vi "FPGA_9505_Thruster_Current_Loop.vi"() -> ()   [LabVIEW 2012]
uses:
  <vilib>/LabVIEW Targets/FPGA/cRIO/cRIO-9505/controls.llb/_nicrio_cRIO-9505_DriveStatus.ctl
  <vilib>/Platform/TimedLoop/XDataNode/timing_clust.ctl
  <vilib>/Platform/TimedLoop/XDataNode/nitl_modes.ctl
  <vilib>/Platform/TimedLoop/XDataNode/wakeup.ctl
  <vilib>/LabVIEW Targets/FPGA/cRIO/cRIO-9505/controls.llb/_nicrio_cRIO-9505_DriveDirection.ctl
  <vilib>/rvi/Emulation/niFpgaSctlEmulationRegisterWithScheduler.vi
  <vilib>/rvi/Emulation/niFpgaSctlEmulationScheduler.vi
  <vilib>/rvi/Emulation/niFpgaSctlEmulationGetInTimedLoop.vi
  <vilib>/rvi/eio/common/nirviEmuTemplateMethod_errors.vi
  <vilib>/rvi/Emulation/niFpgaSctlEmulationGlobalWrite.vi
  <vilib>/rvi/eio/common/nirviEmuTemplatePropertyGet_noerrors.vi
  <vilib>/Platform/TimedLoop/XDataNode/XDataNode.xnode
  <vilib>/eio/EIONode/EIONode.xnode
  <vilib>/eio/EIOMethodNode/EIOMethodNode.xnode
  <vilib>/eio/EIOPropertyNode/EIOPropertyNode.xnode
  <vilib>/rvi/eio/common/nirviEmuTemplatePropertyGet_errors.vi
  <vilib>/rvi/eio/common/nirviEmuTemplatePropertySet_errors.vi
  <vilib>/rvi/eio/common/nirviEmuTemplatePropertySet_noerrors.vi
  <vilib>/Platform/TimedLoop/XDataNode/XDNodeRunTimeDep.lvlib
panel:
  in  "Tab Control":enum32{"Control", "Debugging 1", "Debugging 2"}(tab)
  out "PWM Duty Cycle 3":i16
  in  "Current Loop\nRate (usec) 1":u32=50
  in  "Current Setpoint 1":i16 caption="Setpoint"
  in  "Current Limit 1":i16 caption="Setpoint"
  in  "Current Feedback 1":i16
  in  "Current PI gains 1":T1={"Proportional Gain"=20, "Integral Gain"=10, "Derivative Gain"=0}
  out "PWM Duty Cycle 4":i16
  in  "Current Loop\nRate (usec) 2":u32=50
  in  "Current Setpoint 2":i16 caption="Setpoint"
  in  "Current Limit 2":i16 caption="Setpoint"
  in  "Current Feedback 2":i16
  in  "Current PI gains 2":T1={"Proportional Gain"=20, "Integral Gain"=10, "Derivative Gain"=0}
  out "PWM Loop Counter 1":i32(graph)
  out "Sample Current Loop Counter 1":i32(graph)
  out "Current Sense 1":i16(graph)
  in  "Trig AI 1":bool
  out "PWM Duty Cycle 1":i16(graph)
  out "Current Loop Counter 1":i32(graph)
  out "PWM Loop Counter 2":i32(graph)
  out "PWM Duty Cycle 2":i16(graph)
  out "Current Loop Counter 2":i32(graph)
  in  "Trig AI 2":bool
  out "Current Sense 2":i16(graph)
  out "Sample Current Loop Counter 2":i32(graph)
  out "Vsup Present 2":bool
  out "Drive Fault 2":bool
  out "Drive Status 2":T2
  out "Temp Fault 2":bool
  in  "Enable\nDrive 2":bool
  in  "Disable\nDrive 2":bool
  out "Vsup Present 1":bool
  out "Drive Fault 1":bool
  out "Drive Status 1":T2
  out "Temp Fault 1":bool
  in  "Enable\nDrive 1":bool
  in  "Disable\nDrive 1":bool
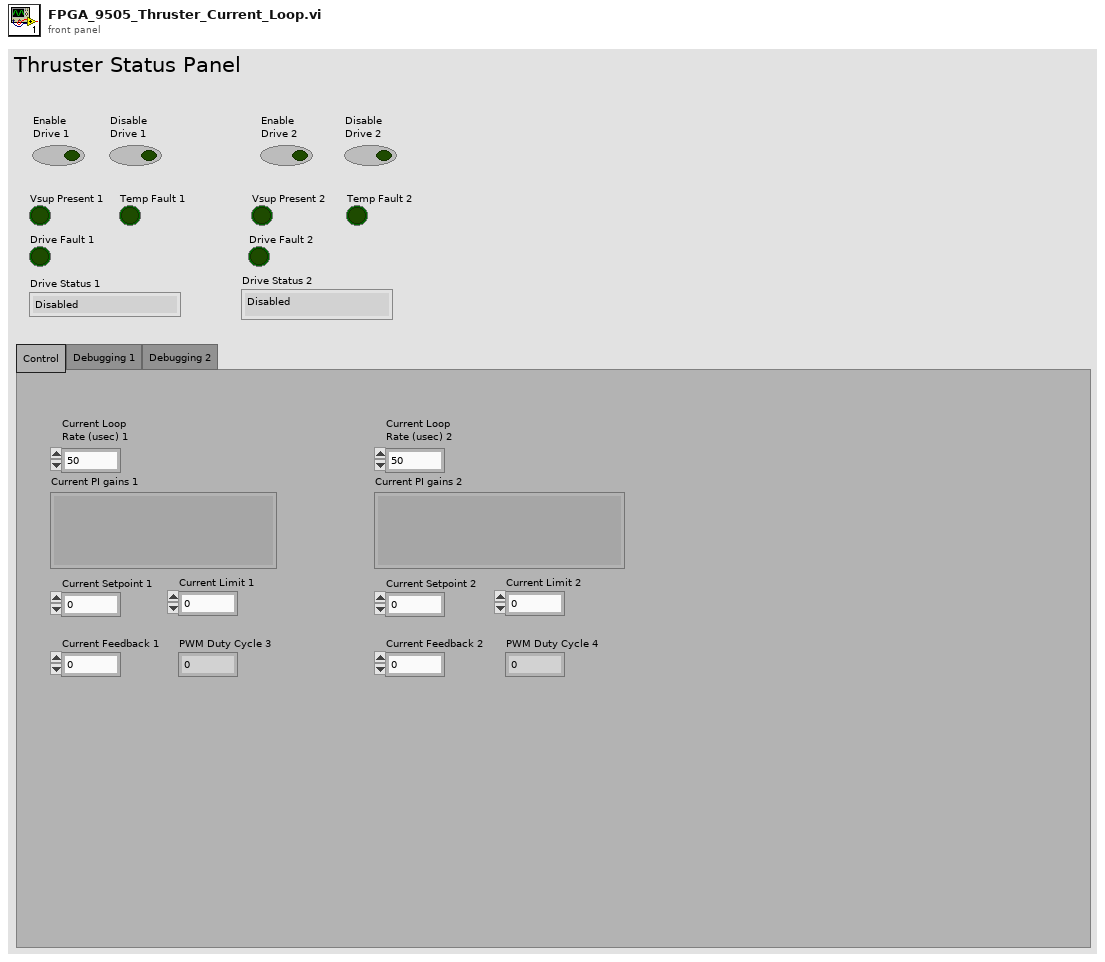
[diagram p1: front panel]
types:
  T1 = cluster{"Proportional Gain":i16, "Integral Gain":i16, "Derivative Gain":i16}
  T2 = typedef "_nicrio_cRIO-9505_DriveStatus.ctl" = enum8{"Enabled", "Disabled", "Disabled by Drive Fault", "Disabled by Temp. Fault", "Disabled by E-Stop", "Unknown"}
  T3 = typedef "XDNodeRunTimeDep.lvlib/timing_clust.ctl" = cluster{"Expected End [f-1]":u64, "Actual End [f-1]":u64, "Finished Late? [f-1]":bool, "Expected End [i-1]":u64, "Actual End [i-1]":u64, "Finished Late? [i-1]":bool, "Expected Start [i]":u64, "Actual Start [i]":u64, "Expected Start [f]":u64, "Actual Start [f]":u64, "Source Name":string, "Structure Name":string, "Period":i64, "Deadline":i64, "Offset":i64, "Start":i64, "Priority":i32, "Timeout":i32, "Mode":T4, "Wakeup Reason":T5, "Error":errorcluster, "Source Type":string, "Secondary Source Type":string, "Global End Time":u64, "Global Start Time":u64, "Frame Duration":u64, "Iteration Duration":u64, "Assigned CPU":i32, "I/O Scan Engine Mode":u32}
  T4 = typedef "XDNodeRunTimeDep.lvlib/nitl_modes.ctl" = enum32{"No Change", "Process missed periods, maintain original phase", "Discard missed periods, maintain original phase", "Process missed periods, ignore original phase", "Discard missed periods, ignore original phase"}
  T5 = typedef "XDNodeRunTimeDep.lvlib/wakeup.ctl" = enum32{"Normal", "Aborted", "Asynchronous wakeup", "Timing source error", "Timed loop error", "Timeout"}
  T6 = typedef "_nicrio_cRIO-9505_DriveDirection.ctl" = enum8{"Clockwise", "Counterclockwise"}
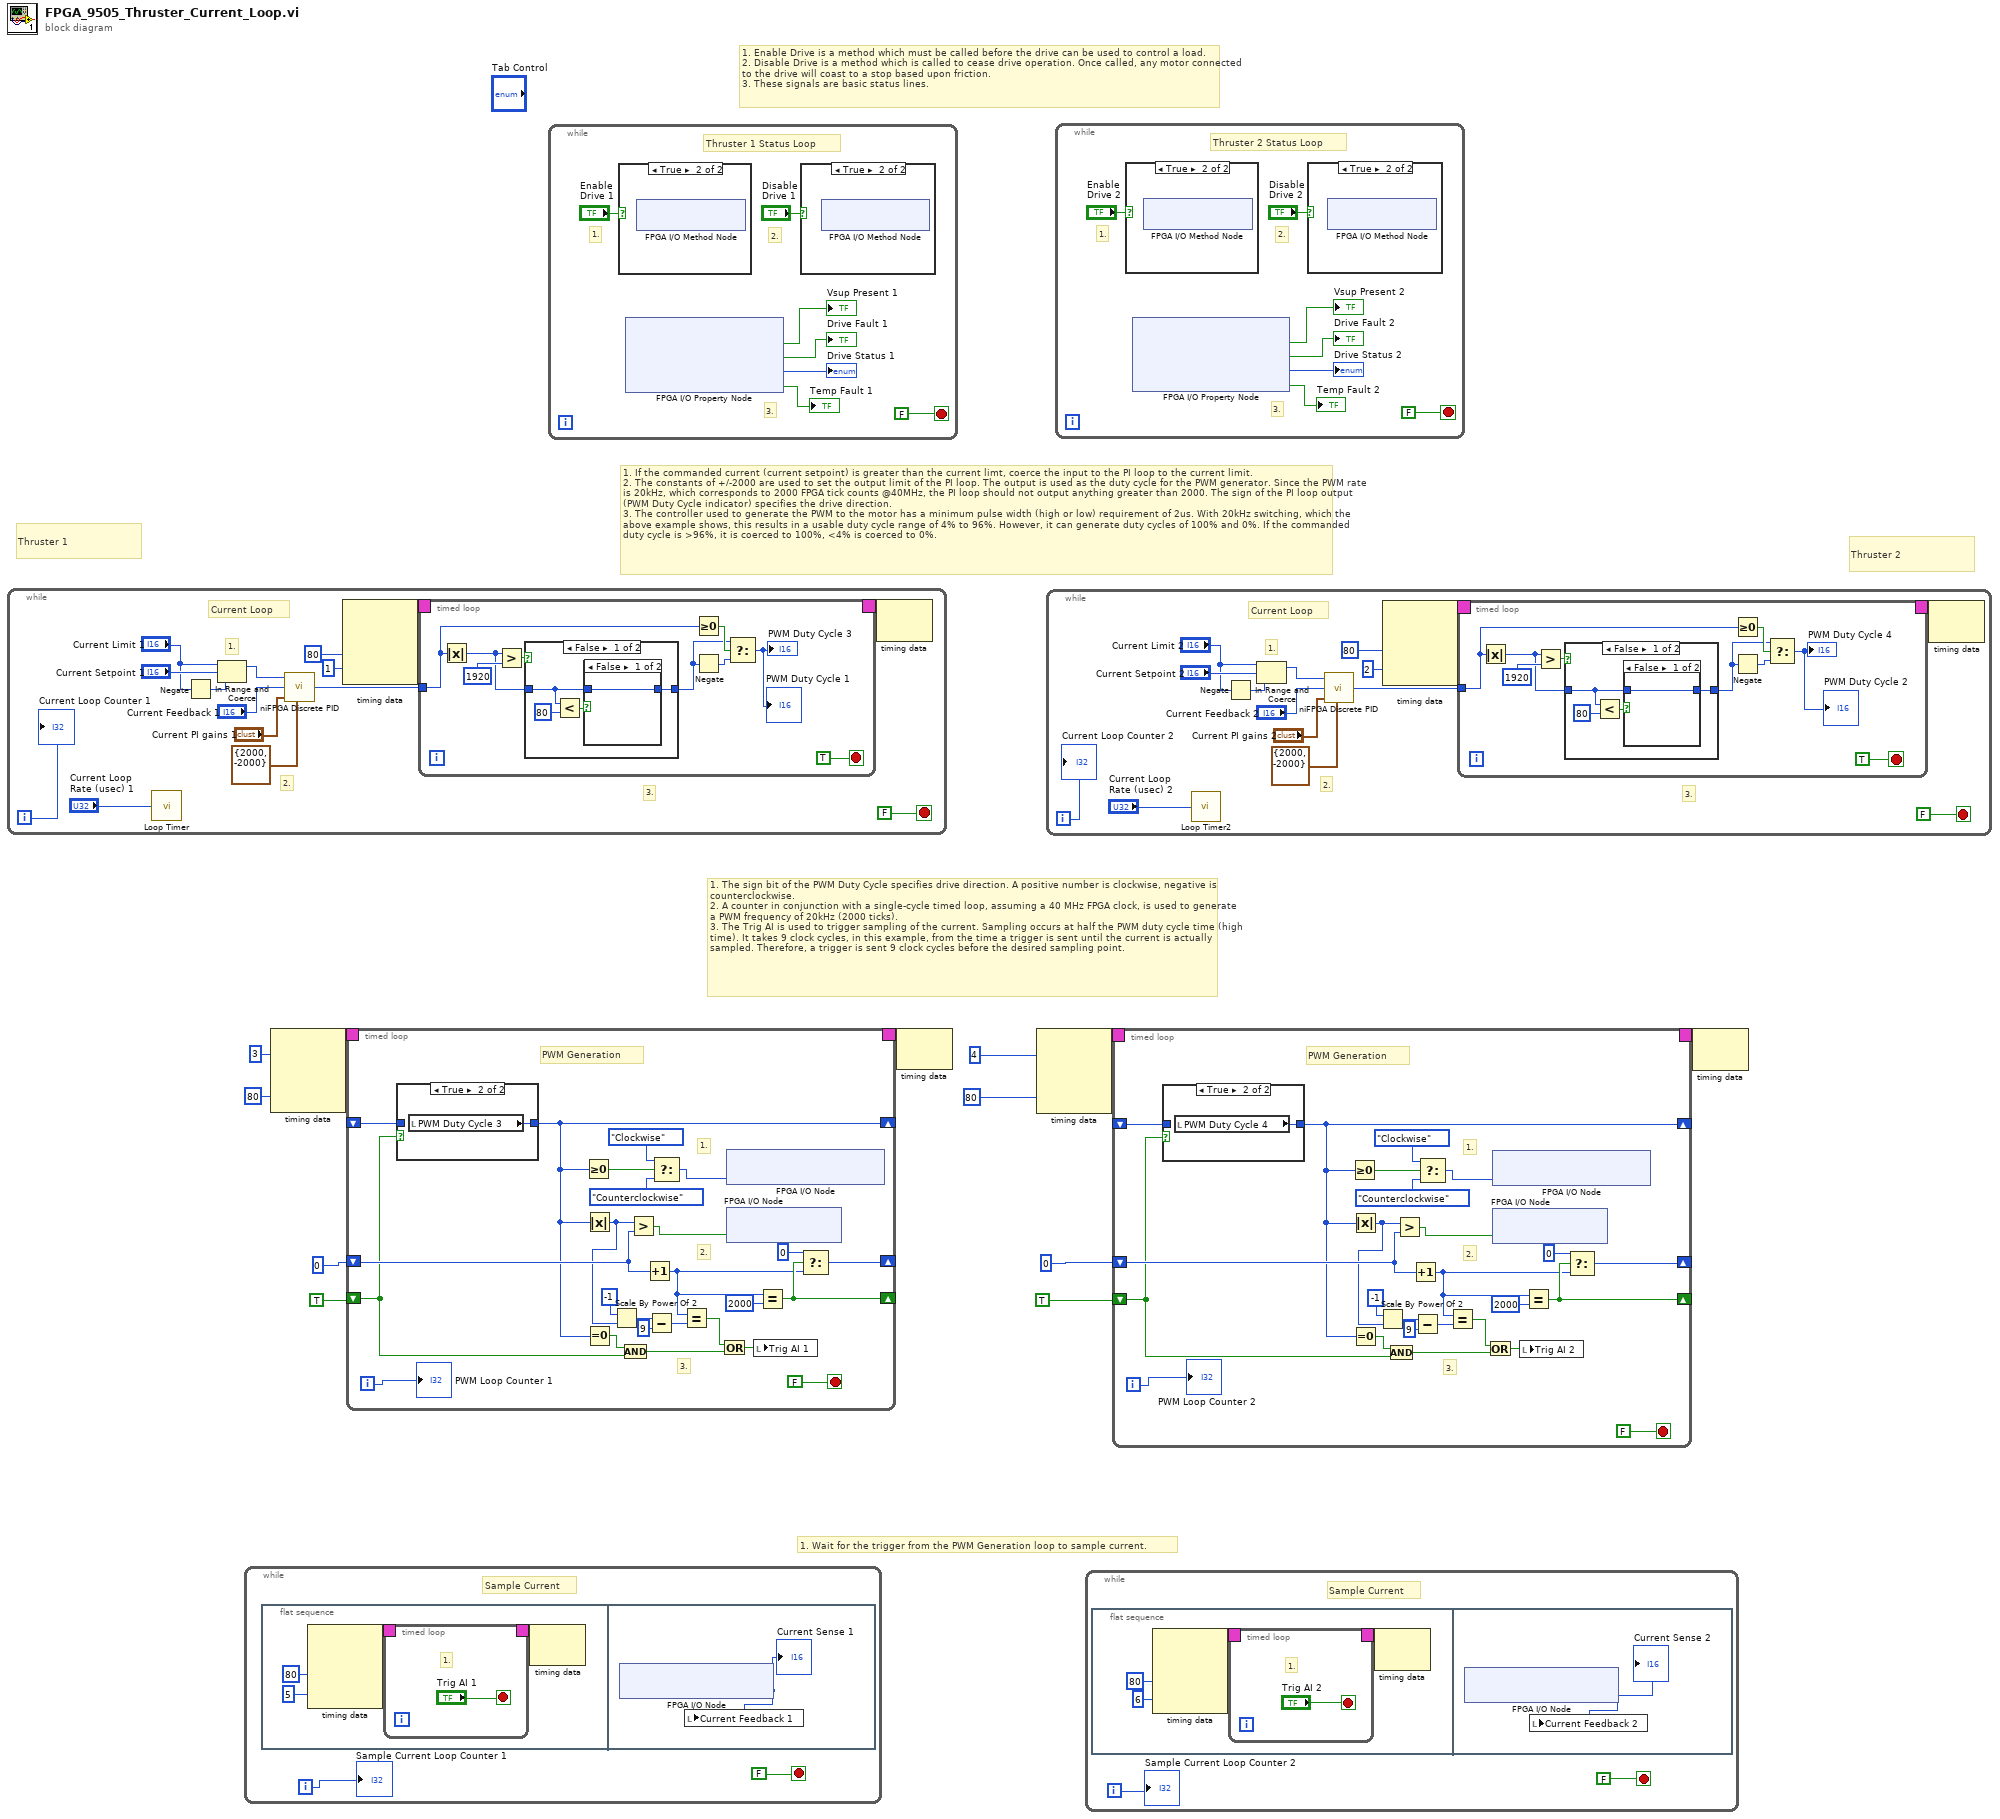
[diagram p0: block diagram]
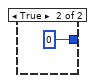
[diagram p4: hidden frame]
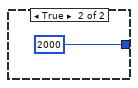
[diagram p5: hidden frame]
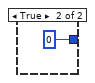
[diagram p6: hidden frame]
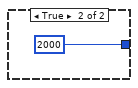
[diagram p7: hidden frame]
diagram:
  # "1. Wait for the trigger from the PWM Generation loop to sample current."
  # "1. The sign bit of the PWM Duty Cycle specifies drive direction. A positive number is clockwise, negative is counterclockwise.\n2. A counter in conjunction with a single-cycle timed loop, assuming a 40 MHz FPGA clock, is used to generate a PWM frequency of 20kHz (2000 ticks).\n3. The Trig AI is used to trigger sampling of the current. Sampling occurs at half the PWM duty cycle time (high time). It takes 9 clock cycles, in this example, from the time a trigger is sent until the current is actually sampled. Therefore, a trigger is sent 9 clock cycles before the desired sampling point."
  # "1. If the commanded current (current setpoint) is greater than the current limt, coerce the input to the PI loop to the current limit.\n2. The constants of +/-2000 are used to set the output limit of the PI loop. The output is used as the duty cycle for the PWM generator. Since the PWM rate is 20kHz, which corresponds to 2000 FPGA tick counts @40MHz, the PI loop should not output anything greater than 2000. The sign of the PI loop output (PWM Duty Cycle indicator) specifies the drive direction.\n3. The controller used to generate the PWM to the motor has a minimum pulse width (high or low) requirement of 2us. With 20kHz switching, which the above example shows, this results in a usable duty cycle range of 4% to 96%. However, it can generate duty cycles of 100% and 0%. If the commanded duty c..."
  # "Thruster 2"
  # "Thruster 1"
  # "1. Enable Drive is a method which must be called before the drive can be used to control a load.\n2. Disable Drive is a method which is called to cease drive operation. Once called, any motor connected to the drive will coast to a stop based upon friction.\n3. These signals are basic status lines."
  n1 = while {
    i -> [w15]
    stop <- FALSE stop-if-true
    # "3."
    # "2."
    # "1."
    # "Current Loop"
    n2 = call "Loop Timer"("Count(uSec)"="Current Loop\nRate (usec) 1") -> ()  [unwired: 1 out]
    n3 = Negate(x="Current Limit 1") -> (-x=w20:i16)
    n4 = In Range and Coerce(upper limit="Current Limit 1", x="Current Setpoint 1", lower limit=w20) -> (coerced(x)=w18:i16)  [unwired: 1 out]
    n5 = call <vilib>:"niFPGA Discrete PID.vi"("setpoint"=w18, "process variable"="Current Feedback 1", "PID gains (x 2^8)"="Current PI gains 1", "output range"=cluster{"output high":i16, "output low":i16} {"output high"=2000, "output low"=-2000}) -> ("output"=w24:i16)  [unwired: 1 in, 4 out]
    n6 = node-c288(80, 1) -> (w23:T3)  [unwired: 2 out]
    n7 = timed-loop {
      timing: w23 -> [_]
      timing-out: [_] -> w22
      tunnel: w24 -> [w30]
      stop <- TRUE stop-if-true
      n8 = Absolute Value(x=w30) -> (abs(x)=w31:i16)
      n9 = Greater?(x=w31, y=i16 1920) -> (0:w33:bool)
      n10 = case shown="False" w33 {
        tunnel: [w39 i16 2000] -> w32
        tunnel: w31 -> [w37 _]
        frame False {
          n11 = Less?(x=w37, y=i16 80) -> (x < y?=w38:bool)
          n12 = case shown="False" w38 {
            tunnel: [w41 i16 0] -> w39
            tunnel: w37 -> [w41 _]
            frame False {
            }
            frame True {
            }
          }
        }
        frame True {
        }
      }
      n13 = Greater Or Equal To 0?(x=w30) -> (x >= 0?=w36:bool)
      n14 = Negate(x=w32) -> (-x=w35:i16)
      n15 = Select(t=w32, s=w36, f=w35) -> (s? t:f=→"PWM Duty Cycle 3" →"PWM Duty Cycle 1":i16)
    }
    n16 = node-c288(w22) -> ()  [unwired: 1 out]
    "Current Loop Counter 1" <- w15
  }
  n17 = while {
    i -> [w51]
    stop <- FALSE stop-if-true
    # "Sample Current"
    n18 = flat-sequence {
      frame #0 {
        n19 = node-c288(80, 5) -> (w56:T3)  [unwired: 2 out]
        n20 = timed-loop {
          timing: w56 -> [_]
          timing-out: [_] -> w55
          stop <- "Trig AI 1" stop-if-true
          # "1."
        }
        n21 = node-c288(w55) -> ()  [unwired: 1 out]
      }
      frame #1 {
        n22 = xnode "FPGA I/O Node"() -> ("Mod2/Current Sense 2"=w65:i16)  [unwired: 1 in, 1 out]
        "Current Sense 1" <- w65
        n23 = local write "Current Feedback 1"(w65) -> ()
      }
    }
    "Sample Current Loop Counter 1" <- w51
  }
  n24 = node-c288(3, 80) -> (w12:T3)  [unwired: 2 in]
  n25 = timed-loop {
    timing: w12 -> [_]
    timing-out: [_] -> w11
    shift-right: [w87] -> _
    shift-left: i16 0 -> [w90]
    shift-right: [w86] -> _
    shift-left: TRUE -> [w83]
    shift-right: [w72] -> _
    shift-left: _ -> [w85]
    i -> [w66]
    stop <- FALSE stop-if-true
    # "3."
    # "2."
    # "1."
    # "PWM Generation"
    n26 = case shown="True" w83 {
      tunnel: [w91 w92] -> w72
      tunnel: w85 -> [w91 _]
      frame False {
      }
      frame True {
        n27 = local read "PWM Duty Cycle 3"() -> (w92:i16)
      }
    }
    n28 = Greater Or Equal To 0?(x=w72) -> (x >= 0?=w79:bool)
    n29 = Absolute Value(x=w72) -> (abs(x)=w70:i16)
    n30 = Equal To 0?(x=w72) -> (x = 0?=w84:bool)
    n31 = Scale By Power Of 2(n=i8 -1, x=w70) -> (x*2^n=w74:i16)
    n32 = And(x=w84, y=w83) -> (x .and. y?=w80:bool)
    n33 = Greater?(x=w70, y=w90) -> (0:w67:bool)
    n34 = Increment(x=w90) -> (x+1=w82:i16)
    n35 = Subtract(x=w74, y=i8 9) -> (x-y=w73:i16)
    n36 = Select(t=_nicrio_cRIO-9505_DriveDirection."Clockwise", s=w79, f=_nicrio_cRIO-9505_DriveDirection."Counterclockwise") -> (s? t:f=w68:T6)
    n37 = Equal?(x=w82, y=w73) -> (x = y?=w81:bool)
    n38 = Or(x=w81, y=w80) -> (x .or. y?=w76:bool)
    n39 = xnode "FPGA I/O Node"("Mod2/Drive Direction 2"=w68) -> ()  [unwired: 1 in, 1 out]
    n40 = xnode "FPGA I/O Node"("Mod2/Motor 2"=w67) -> ()  [unwired: 1 in, 1 out]
    n41 = local write "Trig AI 1"(w76) -> ()
    n42 = Equal?(x=w82, y=i16 2000) -> (x = y?=w86:bool)
    n43 = Select(t=i16 0, s=w86, f=w82) -> (s? t:f=w87:i16)
    "PWM Loop Counter 1" <- w66
  }
  n44 = while {
    stop <- FALSE stop-if-true
    # "3."
    # "2."
    # "1."
    # "Thruster 1 Status Loop"
    n45 = case shown="True" "Enable\nDrive 1" {
      frame False {
      }
      frame True {
        n46 = xnode "FPGA I/O Method Node"() -> ()  [unwired: 1 in, 1 out]
      }
    }
    n47 = xnode "FPGA I/O Property Node"() -> ("Vsup Present"=→"Vsup Present 1":bool, "Drive Fault"=→"Drive Fault 1":bool, "Drive Status"=→"Drive Status 1":T2, "Over Temperature Fault"=→"Temp Fault 1":bool)  [unwired: 1 in, 1 out]
    n48 = case shown="True" "Disable\nDrive 1" {
      frame False {
      }
      frame True {
        n49 = xnode "FPGA I/O Method Node"() -> ()  [unwired: 1 in, 1 out]
      }
    }
  }
  n50 = node-c288(w11) -> ()  [unwired: 1 out]
  n51 = node-c288(4, 80) -> (w6:T3)  [unwired: 2 in]
  n52 = while {
    i -> [w104]
    stop <- FALSE stop-if-true
    # "3."
    # "2."
    # "1."
    # "Current Loop"
    n53 = call "Loop Timer2"("Count(uSec)"="Current Loop\nRate (usec) 2") -> ()  [unwired: 1 out]
    n54 = Negate(x="Current Limit 2") -> (-x=w109:i16)
    n55 = In Range and Coerce(upper limit="Current Limit 2", x="Current Setpoint 2", lower limit=w109) -> (coerced(x)=w107:i16)  [unwired: 1 out]
    n56 = call <vilib>:"niFPGA Discrete PID.vi"("setpoint"=w107, "process variable"="Current Feedback 2", "PID gains (x 2^8)"="Current PI gains 2", "output range"=cluster{"output high":i16, "output low":i16} {"output high"=2000, "output low"=-2000}) -> ("output"=w113:i16)  [unwired: 1 in, 4 out]
    n57 = node-c288(80, 2) -> (w112:T3)  [unwired: 2 out]
    n58 = timed-loop {
      timing: w112 -> [_]
      timing-out: [_] -> w111
      tunnel: w113 -> [w119]
      stop <- TRUE stop-if-true
      n59 = Absolute Value(x=w119) -> (abs(x)=w120:i16)
      n60 = Greater?(x=w120, y=i16 1920) -> (0:w122:bool)
      n61 = case shown="False" w122 {
        tunnel: [w128 i16 2000] -> w121
        tunnel: w120 -> [w126 _]
        frame False {
          n62 = Less?(x=w126, y=i16 80) -> (x < y?=w127:bool)
          n63 = case shown="False" w127 {
            tunnel: [w130 i16 0] -> w128
            tunnel: w126 -> [w130 _]
            frame False {
            }
            frame True {
            }
          }
        }
        frame True {
        }
      }
      n64 = Greater Or Equal To 0?(x=w119) -> (x >= 0?=w125:bool)
      n65 = Negate(x=w121) -> (-x=w124:i16)
      n66 = Select(t=w121, s=w125, f=w124) -> (s? t:f=→"PWM Duty Cycle 4" →"PWM Duty Cycle 2":i16)
    }
    n67 = node-c288(w111) -> ()  [unwired: 1 out]
    "Current Loop Counter 2" <- w104
  }
  n68 = while {
    stop <- FALSE stop-if-true
    # "3."
    # "2."
    # "1."
    # "Thruster 2 Status Loop"
    n69 = case shown="True" "Enable\nDrive 2" {
      frame False {
      }
      frame True {
        n70 = xnode "FPGA I/O Method Node"() -> ()  [unwired: 1 in, 1 out]
      }
    }
    n71 = xnode "FPGA I/O Property Node"() -> ("Vsup Present"=→"Vsup Present 2":bool, "Drive Fault"=→"Drive Fault 2":bool, "Drive Status"=→"Drive Status 2":T2, "Over Temperature Fault"=→"Temp Fault 2":bool)  [unwired: 1 in, 1 out]
    n72 = case shown="True" "Disable\nDrive 2" {
      frame False {
      }
      frame True {
        n73 = xnode "FPGA I/O Method Node"() -> ()  [unwired: 1 in, 1 out]
      }
    }
  }
  n74 = while {
    i -> [w147]
    stop <- FALSE stop-if-true
    # "Sample Current"
    n75 = flat-sequence {
      frame #0 {
        n76 = node-c288(80, 6) -> (w152:T3)  [unwired: 2 out]
        n77 = timed-loop {
          timing: w152 -> [_]
          timing-out: [_] -> w151
          stop <- "Trig AI 2" stop-if-true
          # "1."
        }
        n78 = node-c288(w151) -> ()  [unwired: 1 out]
      }
      frame #1 {
        n79 = xnode "FPGA I/O Node"() -> ("Mod4/Current Sense 2"=w161:i16)  [unwired: 1 in, 1 out]
        "Current Sense 2" <- w161
        n80 = local write "Current Feedback 2"(w161) -> ()
      }
    }
    "Sample Current Loop Counter 2" <- w147
  }
  n81 = timed-loop {
    timing: w6 -> [_]
    timing-out: [_] -> w5
    shift-right: [w183] -> _
    shift-left: i16 0 -> [w186]
    shift-right: [w182] -> _
    shift-left: TRUE -> [w179]
    shift-right: [w168] -> _
    shift-left: _ -> [w181]
    i -> [w162]
    stop <- FALSE stop-if-true
    # "3."
    # "2."
    # "1."
    # "PWM Generation"
    n82 = case shown="True" w179 {
      tunnel: [w187 w188] -> w168
      tunnel: w181 -> [w187 _]
      frame False {
      }
      frame True {
        n83 = local read "PWM Duty Cycle 4"() -> (w188:i16)
      }
    }
    n84 = Greater Or Equal To 0?(x=w168) -> (x >= 0?=w175:bool)
    n85 = Absolute Value(x=w168) -> (abs(x)=w166:i16)
    n86 = Equal To 0?(x=w168) -> (x = 0?=w180:bool)
    n87 = Scale By Power Of 2(n=i8 -1, x=w166) -> (x*2^n=w170:i16)
    n88 = And(x=w180, y=w179) -> (x .and. y?=w176:bool)
    n89 = Greater?(x=w166, y=w186) -> (0:w163:bool)
    n90 = Increment(x=w186) -> (x+1=w178:i16)
    n91 = Subtract(x=w170, y=i8 9) -> (x-y=w169:i16)
    n92 = Select(t=_nicrio_cRIO-9505_DriveDirection."Clockwise", s=w175, f=_nicrio_cRIO-9505_DriveDirection."Counterclockwise") -> (s? t:f=w164:T6)
    n93 = Equal?(x=w178, y=w169) -> (x = y?=w177:bool)
    n94 = Or(x=w177, y=w176) -> (x .or. y?=w172:bool)
    n95 = xnode "FPGA I/O Node"("Mod4/Drive Direction 2"=w164) -> ()  [unwired: 1 in, 1 out]
    n96 = xnode "FPGA I/O Node"("Mod4/Motor 2"=w163) -> ()  [unwired: 1 in, 1 out]
    n97 = local write "Trig AI 2"(w172) -> ()
    n98 = Equal?(x=w178, y=i16 2000) -> (x = y?=w182:bool)
    n99 = Select(t=i16 0, s=w182, f=w178) -> (s? t:f=w183:i16)
    "PWM Loop Counter 2" <- w162
  }
  n100 = node-c288(w5) -> ()  [unwired: 1 out]
